vi "ISX3_Read_Data.vi"(1 "FT_Handle":u32, 2 "Bytes To Read":u32) -> (4 "Handle":u32, 5 "Bytes Read":u32, 6 "Read Data":u8[](array[numeric]))   [LabVIEW 2012, in "Sciospec ISX3 Impedance Analyzer.lvlib"]
uses:
  Sciospec ISX3 Impedance Analyzer.lvlib
panel:
  # "FT_Handle to the USB interface"
  # "FT_Handle to the USB interface"
  # "Number of bytes read from the interface.\nIf an error occurs  while reading from the interface\nthe number differs from \"Bytes To Read\""
  # "Array of data read from the interface."
  # "This VI reads a number of bytes from the USB interface.\nThe USB interfacae (FT_Handle) must be initialized.\nThis VI blocks until the amount of bytes is available"
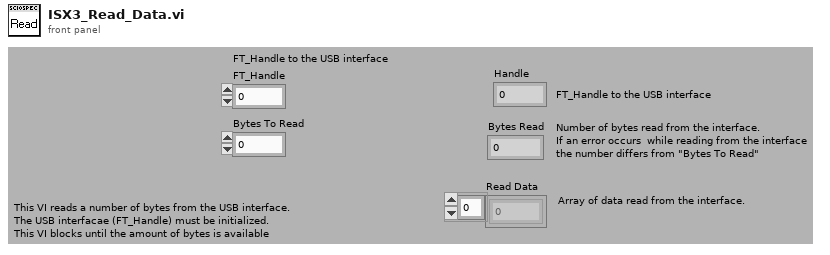
[diagram p1: front panel]
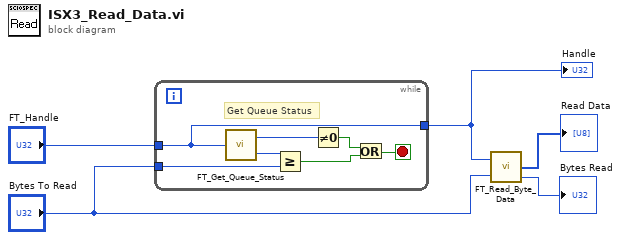
[diagram p0: block diagram]
diagram:
  n1 = while {
    tunnel: "FT_Handle" -> [w8]
    tunnel: "Bytes To Read" -> [w9]
    tunnel: [w8] -> w1
    stop <- w11 stop-if-true
    # "Get Queue Status"
    n2 = call "FT_Get_Queue_Status.vi"("Handle"=w8) -> ("FT_Status"=w7:u32, "Bytes Waiting"=w6:u32)
    n3 = Greater Or Equal?(x=w6, y=w9) -> (x >= y?=w10:bool)
    n4 = Not Equal To 0?(x=w7) -> (x != 0?=w12:bool)
    n5 = Or(x=w12, y=w10) -> (x .or. y?=w11:bool)
  }
  "Handle" <- w1
  n6 = call "FT_Read_Byte_Data.vi"("Handle"=w1, "Bytes To Read"="Bytes To Read") -> ("Read Data"=→"Read Data":u8[], "Bytes Read"=→"Bytes Read":u32)  [unwired: 1 out]
